vi "XY Graph Rebin Plot.vi"(8 "error in (no error)":errorcluster, 9 "Replace Plot (T)?":bool=TRUE, 11 "Selected Plot Info":T1={"Multiplot XY Graph"=refnum, "Mouse Coordinates"={"Horizontal"=0, "Vertical"=0}, "Plot Index"=-1}) -> (0 "Error Out":errorcluster, 1 "Rebinned Plot Message":string, 3 "Rebinned Plot":cluster{"t Array":dbl[], "IRF Array":dbl[]})   [LabVIEW 2021, in "XY Graph Add-Ons.lvlib"]
uses:
  XY Graph Add-Ons.lvlib
  XY Graph Selected Plot Info.ctl
  XY Graph Refnum.ctl
  <vilib>/Utility/miscctls.llb/LVPoint32TypeDef.ctl
  Histograms/Histogram Window.lvlib
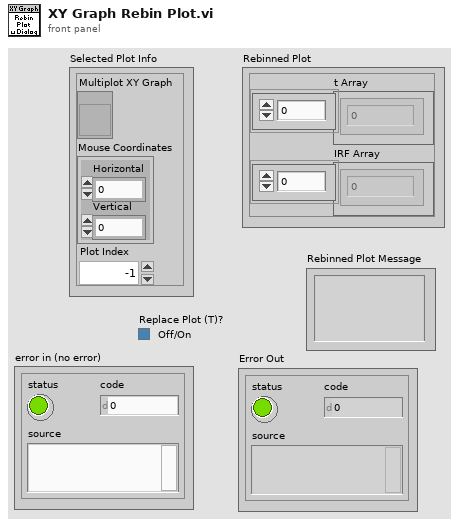
[diagram p1: front panel]
types:
  T1 = typedef "XY Graph Add-Ons.lvlib/XY Graph Selected Plot Info.ctl" = cluster{"Multiplot XY Graph":T2, "Mouse Coordinates":T3, "Plot Index":i32}
  T2 = typedef "XY Graph Add-Ons.lvlib/XY Graph Refnum.ctl" = refnum<vi>
  T3 = typedef "LVPoint32TypeDef.ctl" = cluster{"Horizontal":i32, "Vertical":i32}
  T4 = typedef "XY Graph Add-Ons.lvlib/XY Plot Data.ctl" = cluster{"X Array":dbl[], "Y Array":dbl[]}
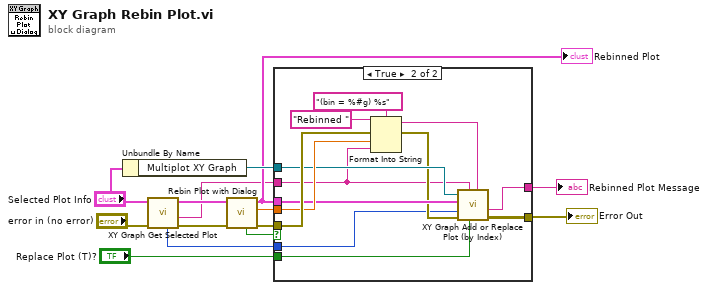
[diagram p0: block diagram]
diagram:
  n1 = Unbundle By Name("Selected Plot Info") -> ("Multiplot XY Graph"=w12:T2)
  n2 = call "XY Graph Get Selected Plot.vi"("error in (no error)"="error in (no error)", "Selected Plot Info"="Selected Plot Info") -> ("error out"=w5:errorcluster, "Plot Name"=w4:string, "Plot"=w6:T4, "Plot Index in (dup)"=w3:i32)  [unwired: 4 in, 2 out]
  n3 = call "Rebin Plot with Dialog.vi"("error in (no error)"=w5, "Original Bin Histogram"=w6) -> ("error out"=w10:errorcluster, "Bin Size_"=w9:dbl, "Rebinned Histogram"=w11:cluster{"Axis":dbl[], "Histogram":dbl[]}, "OK?"=w8:bool)  [unwired: 5 in, 1 out]
  "Rebinned Plot" <- w11
  n4 = case shown="True" w8 {
    tunnel: w3 -> [_ w22]
    tunnel: [_ w16] -> w14
    tunnel: [w15 w17] -> w13
    tunnel: w12 -> [_ w24]
    tunnel: w11 -> [_ w25]
    tunnel: w4 -> [_ w19]
    tunnel: w10 -> [w15 w27]
    tunnel: w9 -> [_ w26]
    tunnel: "Replace Plot (T)?" -> [_ w18]
    frame False {
    }
    frame True {
      n5 = Format Into String(format string="(bin = %#g) %s", initial string="Rebinned ", error in=w27, w26, w19) -> (resulting string=w20:string, error out=w23:errorcluster)
      n6 = call "XY Graph Add or Replace Plot (by Index).vi"("New Plot Name"=w20, "Replace Plot (T)?"=w18, "Original Plot Name"=w19, "error in (no error)"=w23, "Plot Index"=w22, "Plot in"=w25, "XYGraph in"=w24) -> ("error out"=w17:errorcluster, "Message"=w16:string)  [unwired: 3 in]
    }
  }
  "Error Out" <- w13
  "Rebinned Plot Message" <- w14
